vi "test bmp parse.vi"() -> ()   [LabVIEW 2018, in "Data Parser.lvclass"]
uses:
  Data Parser.lvclass
  Bmp data.ctl
panel:
  out "bmp data":T1
  in  "file string":string="<bmp\nname Rudolf\nhead sys/rudolf_f-r\nsmall sys/rudolf_s_x3\nfile(0-69) sys/rudolf-r_0 w 90 h 90 row 10 col 7\nfile(70-139) sys/rudolf-r_1 w 90 h 90 row 10 col 7\nfile(140-149) sys/rudolf-r_2 w 168 h 99 row 5 col 2\nfile(150-155) sys/rudolf-r_3 w 106 h 73 row 6 col 1\nwalking_frame_rate 3\nwalking_speed 6.000000\nwalking_speedz 2.500000\nrunning_frame_rate 3\nrunning_speed 13.000000\nrunning_speedz 1.600000\nheavy_walking_speed 4.200000\nheavy_walking_speedz 1.850000\nheavy_running_speed 7.000000\nheavy_running_speedz 1.000000\njump_height -16.299999\njump_distance 10.000000\njump_distancez 3.750000\ndash_height -10.000000\ndash_distance 18.000000\ndash_distancez 5.000000\nrowing_height -2.000000\nrowing_distance 5.000000\nlimb_head sys/limb_rudolf_head 1000 1000 5 5 0 25\nlimb_chest sys/limb_rudolf_chest 1000 1000 5 5 0 14\nlimb_hip sys/limb_rudolf_chest 1000 1000 5 5 20 17\nlimb_l_hand_a sys/limb_rudolf_hand 1000 1000 5 5 15 5\nlimb_r_hand_a sys/limb_rudolf_hand 1000 1000 5 5 25 4\nlimb_l_hand_b sys/limb_rudolf_hand 500 500 10 10 0 23\nlimb_r_hand_b sys/limb_rudolf_hand 500 500 10 10 30 23\nlimb_l_hand_w sys/limb_rudolf_weapon 1000 1000 5 5 0 5\nlimb_r_hand_w sys/limb_rudolf_weapon 1000 1000 5 5 0 5\nlimb_l_hand_c sys/limb_rudolf_hand_cover 500 500 10 10 0 23\nlimb_r_hand_c sys/limb_rudolf_hand_cover 500 500 10 10 30 23\nlimb_l_leg_a sys/limb_rudolf_leg 500 500 10 10 0 2\nlimb_l_leg_b sys/limb_rudolf_leg 500 500 10 10 10 6\nlimb_r_leg_a sys/limb_rudolf_leg 500 500 10 10 20 2\nlimb_r_leg_b sys/limb_rudolf_leg 500 500 10 10 30 6\nlimb_l_foot sys/limb_rudolf_leg 500 500 10 10 40 14\nlimb_r_foot sys/limb_rudolf_leg 500 500 10 10 60 14\nlimb_effect sys/limb_effect 1000 1000 5 5 0 25\nlimb_effect2 sys/limb_rudolf_effect 500 500 10 10 0 35\nlimb_head_blood 583 846 569 839 570 840 568 843 600 841 597 842 597 842 652 844 652 844 652 844 -1 -1 -1 -1 -1 -1 420 862 420 862 419 862 657 661 597 761 591 761 591 761 619 683 -1 -1 619 683 579 843 579 843 -1 -1 -1 -1 -1 -1 -1 -1 -1 -1\nlimb_hand_weapon 242 326 244 326 420 260 424 258 238 345 221 170 360 247 399 284 228 322 304 342 369 243 230 312 230 320 275 128 345 268 445 218 245 280 313 390 222 131 243 126 238 202 298 155 147 379 291 191 -1 -1 -1 -1 -1 -1 -1 -1 -1 -1 -1 -1 -1 -1 -1 -1 201 162 -1 -1 -1 -1 -1 -1 -1 -1 -1 -1 -1 -1 -1 -1 -1 -1 -1 -1 -1 -1 -1 -1 -1 -1 -1 -1 -1 -1 -1 -1 -1 -1 -1 -1 -1 -1 -1 -1 -1 -1 -1 -1 -1 -1 -1 -1 -1 -1 -1 -1 -1 -1 -1 -1\nresized 3\ndefault_centerx 44\ndefault_centery 84\nbmp>\n<f 0 standing\n   pic 0 wait 5 next 1 centerx 46 hit_Fa 285 hit_Fj 273 hit_Uj 250 hit_Dj 260 hit_ja 295\n   <bp x 48.464444444444446 y 38.35111111111111 bp>\n   <w kind 1 x 51 y 54 weaponact 30 cover 1 w>\n   <b kind 0 x 26 y 23 w 43 h 62 b>\nf>\n\n<f 1 -\n   pic 1 wait 4 next 2 dvz 123 centerx 47 hit_Fa 285 hit_Fj 273 hit_Uj 250 hit_Dj 260 hit_ja 295\n   <bp x 49.464444444444446 y 38.12888888888889 bp>\n   <w kind 1 x 52 y 54 weaponact 30 cover 1 w>\n   <b kind 0 x 26 y 23 w 43 h 62 b>\nf>\n\n<f 2 -\n   pic 2 wait 3 next 3 centerx 47 hit_Fa 285 hit_Fj 273 hit_Uj 250 hit_Dj 260 hit_ja 295\n   <bp x 49.464444444444446 y 37.906666666666666 bp>\n   <w kind 1 x 52 y 53 weaponact 30 cover 1 w>\n   <b kind 0 x 26 y 23 w 43 h 62 b>\nf>\n\n<f 3 -\n   pic 3 wait 8 next 4 hit_Fa 285 hit_Fj 273 hit_Uj 250 hit_Dj 260 hit_ja 295\n   <bp x 46.464444444444446 y 37.684444444444445 bp>\n   <w kind 1 x 49 y 52 weaponact 30 cover 1 w>\n   <b kind 0 x 26 y 23 w 43 h 62 b>\nf>\n\n<f 4 -\n   pic 2 wait 3 next 999 centerx 47 hit_Fa 285 hit_Fj 273 hit_Uj 250 hit_Dj 260 hit_ja 295\n   <bp x 49.464444444444446 y 37.906666666666666 bp>\n   <w kind 1 x 52 y 53 weaponact 30 cover 1 w>\n   <b kind 0 x 26 y 23 w 43 h 62 b>\nf>\n\n<f 5 walking\n   pic 4 state 1 wait 3 next 999 centerx 46 centery 83 hit_Fa 285 hit_Fj 273 hit_Uj 250 hit_Dj 260 hit_ja 295\n   <bp x 48.464444444444446 y 37.79555555555555 bp>\n   <w kind 1 x 49 y 51 weaponact 30 cover 1 w>\n   <i kind 1 x 45 y 21 w 25 h 65 catchingact 120 120 caughtact 130 130 i>\n   <b kind 0 x 27 y 18 w 34 h 64 b>\nf>\n\n<f 6 -\n   pic 5 state 1 wait 3 next 999 centerx 45 hit_Fa 285 hit_Fj 273 hit_Uj 250 hit_Dj 260 hit_ja 295\n   <bp x 47.464444444444446 y 38.79555555555555 bp>\n   <w kind 1 x 48 y 51 weaponact 30 cover 1 w>\n   <i kind 1 x 45 y 21 w 25 h 65 catchingact 120 120 caughtact 130 130 i>\n   <b kind 0 x 28 y 17 w 33 h 67 b>\nf>\n\n<f 7 -\n   pic 6 state 1 wait 3 next 999 centerx 47 hit_Fa 285 hit_Fj 273 hit_Uj 250 hit_Dj 260 hit_ja 295\n   <bp x 49.464444444444446 y 38.57333333333334 bp>\n   <w kind 1 x 50 y 51 weaponact 30 cover 1 w>\n   <i kind 1 x 45 y 21 w 25 h 65 catchingact 120 120 caughtact 130 130 i>\n   <b kind 0 x 29 y 16 w 34 h 67 b>\nf>\n\n<f 8 -\n   pic 7 state 1 wait 3 next 999 centerx 48 centery 83 hit_Fa 285 hit_Fj 273 hit_Uj 250 hit_Dj 260 hit_ja 295\n   <bp x 50.464444444444446 y 37.79555555555555 bp>\n   <w kind 1 x 52 y 51 weaponact 30 cover 1 w>\n   <i kind 1 x 45 y 21 w 25 h 65 catchingact 120 120 caughtact 130 130 i>\n   <b kind 0 x 31 y 17 w 34 h 65 b>\nf>\n\n<f 9 running\n   pic 20 state 2 wait 3 centerx 37\n   sound mp3/003\n   <bp x 65.5137545143159 y 55.18645971015323 bp>\n   <w kind 1 x 51 y 59 weaponact 32 cover 1 w>\n   <b kind 0 x 30 y 24 w 38 h 60 b>\nf>\n\n<f 10 -\n   pic 21 state 2 wait 3 centerx 37\n   <bp x 65.5137545143159 y 56.29757082126433 bp>\n   <w kind 1 x 51 y 60 weaponact 32 cover 1 w>\n   <b kind 0 x 30 y 24 w 38 h 60 b>\nf>\n\n<f 11 -\n   pic 22 state 2 wait 3 centerx 37\n   sound mp3/004\n   <bp x 65.5137545143159 y 55.18645971015323 bp>\n   <w kind 1 x 51 y 61 weaponact 32 cover 1 w>\n   <b kind 0 x 30 y 24 w 38 h 60 b>\nf>\n\n<f 12 heavy_obj_walk\n   pic 23 state 1 wait 3 centerx 45\n   <bp x 46.79777777777778 y 39.24 bp>\n   <w kind 1 x 42.22222222222222 y 24.875555555555557 weaponact 10 w>\n   <b kind 0 x 26 y 17 w 38 h 71 b>\nf>\n\n<f 13 -\n   pic 24 state 1 wait 3\n   <bp x 45.79777777777778 y 39.01777777777778 bp>\n   <w kind 1 x 41.22222222222222 y 24.653333333333336 weaponact 10 w>\n   <b kind 0 x 27 y 18 w 36 h 69 b>\nf>\n\n<f 14 -\n   pic 25 state 1 wait 3 centerx 46\n   <bp x 47.79777777777778 y 39.01777777777778 bp>\n   <w kind 1 x 43.22222222222222 y 24.653333333333336 weaponact 10 w>\n   <b kind 0 x 27 y 16 w 38 h 70 b>\nf>\n\n<f 15 -\n   pic 26 state 1 wait 3 centerx 48\n   <bp x 49.79777777777778 y 38.79555555555555 bp>\n   <w kind 1 x 45.22222222222222 y 24.431111111111115 weaponact 10 w>\n   <b kind 0 x 29 y 16 w 38 h 72 b>\nf>\n\n<f 16 heavy_obj_run\n   pic 125 state 2 wait 3 centerx 40\n   sound mp3/003\n   <bp x 41.79777777777778 y 38.79555555555555 bp>\n   <w kind 1 x 37.22222222222222 y 24.431111111111115 weaponact 10 w>\n   <b kind 0 x 27 y 15 w 30 h 68 b>\nf>\n\n<f 17 -\n   pic 126 state 2 wait 3\n   <bp x 45.79777777777778 y 38.35111111111111 bp>\n   <w kind 1 x 41.22222222222222 y 23.986666666666665 weaponact 10 w>\n   <b kind 0 x 33 y 15 w 31 h 68 b>\nf>\n\n<f 18 -\n   pic 127 state 2 wait 3 centerx 46\n   sound mp3/004\n   <bp x 47.79777777777778 y 38.79555555555555 bp>\n   <w kind 1 x 43.22222222222222 y 24.653333333333336 weaponact 10 w>\n   <b kind 0 x 29 y 20 w 37 h 63 b>\nf>\n\n<f 19 heavy_stop_run\n   pic 128 state 15 wait 7 next 999 dvx 2 centerx 38\n   sound mp3/009\n   <bp x 41.32306886667164 y 39.190553757669235 bp>\n   <w kind 1 x 38.8899896983711 y 24.335554073121564 weaponact 10 w>\n   <b kind 0 x 23 y 21 w 38 h 63 b>\nf>\n\n<f 20 normal_weapon_atck\n   pic 70 state 3 wait 1 next 21 centerx 38\n   <bp x 39.8 y 37.82222222222222 bp>\n   <w kind 1 x 26.592545073322224 y 22.254645252289063 weaponact 31 w>\n   <b kind 0 x 26 y 19 w 34 h 65 b>\nf>\n\n<f 21 -\n   pic 71 state 3 wait 1 next 22 centerx 38\n   sound mp3/008\n   <bp x 43.62444444444444 y 37.92444444444445 bp>\n   <w kind 1 x 41.63440528554246 y 21.504109467745614 weaponact 32 w>\n   <b kind 0 x 29 y 17 w 28 h 67 b>\nf>\n\n<f 22 -\n   pic 72 state 3 wait 1 next 23 centerx 33\n   <bp x 44.08982646609609 y 39.58924737843303 bp>\n   <w kind 1 x 49.32160589714093 y 59.440946875407946 weaponact 24 attacking 1 w>\n   <b kind 0 x 12 y 17 w 40 h 68 b>\nf>\n\n<f 23 -\n   pic 73 state 3 wait 1 next 999 centerx 33 centery 85\n   <bp x 46.58183747280419 y 41.68501265613956 bp>\n   <w kind 1 x 41.82331609590126 y 64.18428829073993 weaponact 25 w>\n   <b kind 0 x 14 y 17 w 34 h 69 b>\n   <b kind 0 x 30 y 66 w 17 h 18 b>\nf>\n\n<f 25 normal_weapon_atck\n   pic 74 state 3 wait 1 next 26 centerx 41\n   <bp x 50.17696571753358 y 39.06775950420733 bp>\n   <w kind 1 x 52 y 51 weaponact 33 cover 1 w>\n   <b kind 0 x 24 y 13 w 33 h 72 b>\nf>\n\n<f 26 -\n   pic 75 state 3 wait 1 next 27 centerx 41\n   sound mp3/008\n   <bp x 49.07477201946767 y 38.68260033531007 bp>\n   <w kind 1 x 58 y 47 weaponact 32 cover 1 w>\n   <b kind 0 x 29 y 17 w 27 h 67 b>\nf>\n\n<f 27 -\n   pic 76 state 3 wait 1 next 28 centerx 33\n   <bp x 39.39302438590751 y 39.56103447170426 bp>\n   <w kind 1 x 50.64327642640106 y 56.22124561746575 weaponact 24 attacking 1 w>\n   <b kind 0 x 14 y 20 w 32 h 64 b>\nf>\n\n<f 28 -\n   pic 77 state 3 wait 1 next 999\n   <bp x 56.25248349990373 y 42.434129183191274 bp>\n   <w kind 1 x 26.13347160923185 y 54.783390010013164 weaponact 25 w>\n   <b kind 0 x 29 y 23 w 32 h 60 b>\nf>\n\n<f 30 jump_weapon_atck\n   pic 80 state 3 wait 1 next 31 centerx 29 centery 89\n   <bp x 41.46019077473909 y 38.358365142781864 bp>\n   <w kind 1 x 29.95234256553649 y 21.49551402119002 weaponact 32 w>\n   <b kind 0 x 21 y 18 w 28 h 58 b>\nf>\n\n<f 31 -\n   pic 81 state 3 wait 1 next 32 centerx 27 centery 90\n   sound mp3/008\n   <bp x 42.49276045988708 y 39.645255650438315 bp>\n   <w kind 1 x 42.23001532517321 y 23.106857251707368 weaponact 33 attacking 2 w>\n   <b kind 0 x 28 y 15 w 23 h 45 b>\n   <b kind 0 x 18 y 43 w 24 h 33 b>\nf>\n\n<f 32 -\n   pic 82 state 3 wait 1 next 33 centerx 25 centery 91\n   <bp x 44.97871535498498 y 41.478136267321915 bp>\n   <w kind 1 x 50.97547888680435 y 60.889746033215864 weaponact 24 attacking 2 w>\n   <b kind 0 x 16 y 37 w 33 h 43 b>\n   <b kind 0 x 34 y 17 w 26 h 38 b>\nf>\n\n<f 33 -\n   pic 83 state 3 wait 4 next 999 centerx 27 centery 92\n   <bp x 47.24850413947085 y 43.129457100584006 bp>\n   <w kind 1 x 42.489982762567934 y 65.62873273518439 weaponact 25 attacking 2 w>\n   <b kind 0 x 16 y 37 w 33 h 43 b>\n   <b kind 0 x 31 y 14 w 26 h 37 b>\nf>\n\n<f 35 run_weapon_atck\n   pic 71 state 3 wait 1 next 36 dvx 6 centerx 45\n   <bp x 43.62444444444444 y 37.92444444444445 bp>\n   <w kind 1 x 41.63440528554246 y 21.504109467745614 weaponact 32 w>\n   <b kind 0 x 26 y 20 w 31 h 65 b>\nf>\n\n<f 36 -\n   pic 72 state 3 wait 1 next 37 dvx 4 centerx 31\n   sound mp3/008\n   <bp x 44.08982646609609 y 39.58924737843303 bp>\n   <w kind 1 x 49.32160589714093 y 58.440946875407946 weaponact 23 attacking 3 w>\n   <b kind 0 x 20 y 20 w 29 h 63 b>\nf>\n\n<f 37 -\n   pic 73 wait 6 next 999 centerx 29\n   <bp x 46.58183747280419 y 41.68501265613956 bp>\n   <w kind 1 x 42.82331609590126 y 64.18428829073993 weaponact 24 attacking 3 w>\n   <b kind 0 x 22 y 22 w 26 h 61 b>\nf>\n\n<f 40 dash_weapon_atck\n   pic 80 state 3 wait 1 next 41 centerx 26 centery 82\n   <bp x 41.46019077473909 y 38.358365142781864 bp>\n   <w kind 1 x 29.95234256553649 y 21.49551402119002 weaponact 31 w>\n   <b kind 0 x 20 y 20 w 27 h 56 b>\nf>\n\n<f 41 -\n   pic 81 state 3 wait 1 next 42 centerx 25 centery 83\n   sound mp3/008\n   <bp x 42.49276045988708 y 39.645255650438315 bp>\n   <w kind 1 x 42.23001532517321 y 23.106857251707368 weaponact 33 attacking 4 w>\n   <b kind 0 x 13 y 37 w 33 h 45 b>\n   <b kind 0 x 28 y 13 w 34 h 33 b>\nf>\n\n<f 42 -\n   pic 82 state 3 wait 1 next 43 centerx 23 centery 83\n   <bp x 44.97871535498498 y 41.478136267321915 bp>\n   <w kind 1 x 51.97547888680435 y 60.889746033215864 weaponact 24 attacking 4 w>\n   <b kind 0 x 13 y 37 w 33 h 45 b>\n   <b kind 0 x 32 y 18 w 30 h 33 b>\nf>\n\n<f 43 -\n   pic 83 state 3 wait 8 next 999 centerx 25\n   <bp x 47.24850413947085 y 43.129457100584006 bp>\n   <w kind 1 x 42.489982762567934 y 64.62873273518439 weaponact 25 attacking 4 w>\n   <b kind 0 x 13 y 37 w 33 h 45 b>\n   <b kind 0 x 28 y 18 w 31 h 37 b>\nf>\n\n<f 45 light_weapon_thw\n   pic 94 state 15 wait 3 next 46\n   <bp x 44.846666666666664 y 38.59111111111111 bp>\n   <w kind 1 x 42.85662750776468 y 22.17077613441228 weaponact 32 w>\n   <b kind 0 x 24 y 20 w 34 h 65 b>\nf>\n\n<f 46 -\n   pic 95 state 15 wait 1 next 47 centerx 42\n   sound mp3/008\n   <bp x 49.31204868831831 y 40.478136267321915 bp>\n   <w kind 1 x 58.535850652335206 y 58.54142301823171 weaponact 22 w>\n   <b kind 0 x 29 y 27 w 32 h 57 b>\nf>\n\n<f 47 -\n   pic 96 state 15 wait 9 next 999 centerx 35\n   <w kind 1 x 107 y 65 weaponact 35 dvx 19 dvy -4 dvz 3 w>\n   <b kind 0 x 15 y 43 w 54 h 21 b>\n   <b kind 0 x 31 y 60 w 32 h 26 b>\nf>\n\n<f 50 heavy_weapon_thw\n   pic 27 state 15 wait 4 next 51\n   <bp x 44.53670834964537 y 38.96496959566491 bp>\n   <w kind 1 x 39.986319716818436 y 25.419297977363684 weaponact 10 w>\n   <b kind 0 x 23 y 19 w 37 h 66 b>\nf>\n\n<f 51 -\n   pic 28 state 15 wait 7 next 999 centerx 39\n   sound mp3/007\n   <w kind 1 x 104 y 47 weaponact 10 dvx 9 dvy -4 dvz 2 w>\n   <b kind 0 x 13 y 44 w 61 h 23 b>\n   <b kind 0 x 26 y 27 w 39 h 57 b>\nf>\n\n<f 52 sky_lgt_wp_thw\n   pic 97 state 15 wait 3 next 53 centerx 29 centery 76\n   <bp x 44.46019077473909 y 32.35836514278185 bp>\n   <w kind 1 x 32.9523425655365 y 14.49551402119002 weaponact 31 w>\n   <b kind 0 x 26 y 17 w 34 h 52 b>\nf>\n\n<f 53 -\n   pic 98 state 15 wait 1 next 54 dvy -2 centerx 30 centery 77\n   sound mp3/008\n   <bp x 47.49276045988708 y 33.64525565043831 bp>\n   <w kind 1 x 47.23001532517321 y 17.106857251707368 weaponact 34 w>\n   <b kind 0 x 25 y 12 w 31 h 66 b>\nf>\n\n<f 54 -\n   pic 99 state 15 wait 9 next 999 centerx 33 centery 76\n   <w kind 1 x 80 y 70 weaponact 23 dvx 16 dvy 8 dvz 3 w>\n   <b kind 0 x 32 y 27 w 36 h 34 b>\n   <b kind 0 x 8 y 42 w 34 h 26 b>\nf>\n\n<f 55 weapon_drink\n   pic 105 state 17 wait 3 next 56 centerx 45 hit_d 999\n   sound mp3/042\n   <w kind 1 x 62.950240476147165 y 27.81086947083836 weaponact 31 w>\n   <b kind 0 x 20 y 17 w 37 h 67 b>\nf>\n\n<f 56 -\n   pic 106 state 17 wait 3 next 57 centerx 45 hit_d 999\n   <w kind 1 x 62.80507006707795 y 26.583434474775675 weaponact 31 w>\n   <b kind 0 x 21 y 25 w 36 h 59 b>\nf>\n\n<f 57 -\n   pic 107 state 17 wait 3 next 58 centerx 45 hit_d 999\n   <w kind 1 x 62.80507006707795 y 25.91676780810901 weaponact 31 w>\n   <b kind 0 x 22 y 22 w 32 h 63 b>\nf>\n\n<f 58 -\n   pic 106 state 17 wait 3 next 55 centerx 45 hit_d 999\n   <w kind 1 x 62.80507006707795 y 26.583434474775675 weaponact 31 w>\n   <b kind 0 x 21 y 18 w 36 h 65 b>\nf>\n\n<f 59 punch\n   pic 13 state 3 wait 4 next 999 centerx 46\n   <bp x 51.45702584630638 y 39.20820242827308 bp>\n   <b kind 0 x 29 y 18 w 33 h 66 b>\nf>\n\n<f 60 -\n   pic 10 state 3 wait 3 next 61 centerx 45 mp 15\n   <bp x 48.75061461791846 y 38.42940829813039 bp>\n   <i kind 2 x 26 y 62 w 37 h 24 vrest 1 i>\n   <b kind 0 x 28 y 20 w 31 h 63 b>\nf>\n\n<f 61 -\n   pic 11 state 3 wait 2 next 62 centerx 47\n   sound mp3/007\n   <bp x 51.18 y 38.59111111111111 bp>\n   <b kind 0 x 33 y 19 w 29 h 63 b>\nf>\n\n<f 62 -\n   pic 12 state 3 wait 1 next 63 centerx 45\n   <o kind 1 x 80 y 62 action 40 dvx 19 dvy -3 oid 202 o>\n   <bp x 49.825838059315736 y 38.98216753134385 bp>\n   <b kind 0 x 31 y 21 w 30 h 64 b>\nf>\n\n<f 63 -\n   pic 13 state 3 wait 4 next 999 centerx 46 hit_a 64\n   <bp x 51.45702584630638 y 39.20820242827308 bp>\n   <b kind 0 x 28 y 17 w 32 h 69 b>\nf>\n\n<f 64 -\n   pic 14 state 3 wait 2 next 66 centerx 47 mp 15\n   <bp x 51.18 y 38.59111111111111 bp>\n   <b kind 0 x 29 y 17 w 30 h 66 b>\nf>\n\n<f 65 -\n   pic 10 state 3 wait 3 next 61 centerx 45 mp 15\n   <bp x 48.75061461791846 y 38.42940829813039 bp>\n   <i kind 2 x 26 y 62 w 37 h 24 vrest 1 i>\n   <b kind 0 x 27 y 23 w 32 h 60 b>\nf>\n\n<f 66 -\n   pic 15 state 3 wait 3 next 67 centerx 45\n   <o kind 1 x 80 y 62 action 40 dvx 18 dvy -2 oid 202 o>\n   <bp x 50.45702584630638 y 39.20820242827308 bp>\n   <b kind 0 x 29 y 20 w 30 h 65 b>\nf>\n\n<f 67 -\n   pic 13 state 3 wait 1 next 999 centerx 46 hit_a 68\n   <bp x 51.45702584630638 y 39.20820242827308 bp>\n   <b kind 0 x 33 y 20 w 27 h 64 b>\nf>\n\n<f 68 -\n   pic 14 state 3 wait 2 next 69 centerx 47 mp 15\n   <bp x 51.18 y 38.59111111111111 bp>\n   <b kind 0 x 32 y 20 w 32 h 62 b>\nf>\n\n<f 69 -\n   pic 12 state 3 wait 2 next 59 centerx 45\n   <o kind 1 x 80 y 62 action 40 dvx 17 dvy -1 oid 202 o>\n   <bp x 49.825838059315736 y 38.98216753134385 bp>\n   <b kind 0 x 30 y 18 w 32 h 66 b>\nf>\n\n<f 70 super_punch\n   pic 132 state 3 wait 1 next 71 centerx 35\n   <bp x 39.18 y 39.257777777777775 bp>\n   <b kind 0 x 19 y 19 w 30 h 66 b>\nf>\n\n<f 71 -\n   pic 133 state 3 wait 2 next 72 dvx 4 centerx 32\n   sound mp3/028\n   <bp x 37.78915887559496 y 40.08682004994553 bp>\n   <i kind 0 x 50 y 14 w 36 h 51 dvx -3 dvy -4 fall 1 injury 10 effect 1 i>\n   <b kind 0 x 9 y 21 w 39 h 61 b>\nf>\n\n<f 72 -\n   pic 134 state 3 wait 1 next 73\n   <i kind 0 x 4 y 11 w 76 h 36 dvx -3 dvy -4 fall 1 injury 10 effect 1 i>\n   <b kind 0 x 27 y 22 w 28 h 62 b>\nf>\n\n<f 73 -\n   pic 135 state 3 wait 1 next 74 centerx 50\n   <b kind 0 x 31 y 19 w 31 h 64 b>\nf>\n\n<f 74 -\n   pic 136 state 3 wait 2 next 75 centerx 37\n   sound mp3/029\n   <bp x 40.933663000829135 y 40.21290188827957 bp>\n   <i kind 0 x 51 y 18 w 32 h 64 dvx 7 dvy -4 fall 70 bdefend 60 injury 65 effect 1 i>\n   <b kind 0 x 18 y 19 w 29 h 64 b>\nf>\n\n<f 75 -\n   pic 137 state 3 wait 1 next 76 centerx 43 centery 82\n   <bp x 45.328713933213194 y 38.15890324252262 bp>\n   <i kind 0 x 5 y 52 w 62 h 31 dvx 7 dvy -4 fall 70 bdefend 60 injury 65 effect 1 i>\n   <b kind 0 x 19 y 14 w 39 h 70 b>\nf>\n\n<f 76 -\n   pic 138 state 3 wait 1 next 77 centerx 49 centery 81\n   <bp x 51.10649171099097 y 37.15890324252262 bp>\n   <b kind 0 x 27 y 16 w 39 h 67 b>\nf>\n\n<f 77 -\n   pic 139 state 3 wait 2 next 78 centerx 55 centery 83\n   <bp x 56.88426948876875 y 39.15890324252262 bp>\n   <b kind 0 x 32 y 18 w 39 h 66 b>\nf>\n\n<f 78 -\n   pic 129 state 3 wait 2 next 79 centerx 48 centery 83\n   <b kind 0 x 27 y 22 w 46 h 63 b>\nf>\n\n<f 79 -\n   pic 119 state 3 wait 3 next 999 centerx 47 centery 83\n   sound mp3/027\n   <bp x 54.268509856829496 y 38.507330714964766 bp>\n   <b kind 0 x 26 y 20 w 42 h 64 b>\nf>\n\n<f 80 jump_attack\n   pic 67 state 3 wait 1 next 81 centerx 38 centery 83\n   <bp x 42.18 y 38.257777777777775 bp>\n   <b kind 0 x 32 y 17 w 30 h 63 b>\nf>\n\n<f 81 -\n   pic 68 state 3 wait 1 next 82 centerx 34 centery 83\n   sound mp3/028\n   <bp x 39.78915887559496 y 39.08682004994553 bp>\n   <i kind 0 x 43 y 13 w 53 h 40 dvx -2 dvy -2 fall 20 arest 15 bdefend 60 injury 35 effect 1 i>\n   <b kind 0 x 24 y 20 w 34 h 60 b>\nf>\n\n<f 82 -\n   pic 69 state 3 wait 1 next 83 centerx 43 centery 82\n   <i kind 0 x 11 y 7 w 75 h 22 dvx -2 dvy -2 fall 20 arest 15 bdefend 60 injury 35 effect 1 i>\n   <b kind 0 x 31 y 18 w 32 h 64 b>\nf>\n\n<f 83 -\n   pic 29 state 3 wait 1 next 84 centerx 51 centery 82\n   <b kind 0 x 38 y 11 w 35 h 70 b>\nf>\n\n<f 84 -\n   pic 39 state 3 wait 1 next 118 centerx 41\n   sound mp3/029\n   <bp x 44.933663000829135 y 40.21290188827957 bp>\n   <i kind 0 x 58 y 11 w 37 h 62 dvx 1 fall 60 arest 15 bdefend 60 injury 35 effect 1 i>\n   <b kind 0 x 26 y 13 w 34 h 67 b>\nf>\n\n<f 85 run_attack\n   pic 140 state 3 wait 1 next 86 dvx 12 centerx 45 centery 90\n   <bp x 73.51375451431592 y 61.18645971015323 bp>\n   <b kind 0 x 30 y 39 w 50 h 52 b>\nf>\n\n<f 86 -\n   pic 141 state 3 wait 1 next 87 dvx 12 centerx 37 centery 90\n   sound mp3/029\n   <i kind 0 x 65 y 36 w 66 h 48 dvx -4 dvy -4 injury 45 effect 1 i>\n   <b kind 0 x 23 y 38 w 49 h 51 b>\nf>\n\n<f 87 -\n   pic 142 state 3 wait 1 next 88 centerx 48 centery 90\n   sound mp3/028\n   <bp x 75.91504918785502 y 61.27127540437745 bp>\n   <i kind 0 x 65 y 36 w 66 h 48 dvx -4 dvy -4 injury 45 effect 1 i>\n   <b kind 0 x 30 y 39 w 51 h 48 b>\nf>\n\n<f 88 -\n   pic 143 state 3 wait 1 next 89 centerx 53 centery 90\n   <bp x 80.47060474341058 y 60.82683095993299 bp>\n   <i kind 0 x 22 y 35 w 81 h 53 dvx 10 dvy -7 fall 70 vrest 15 bdefend 60 injury 35 effect 1 i>\n   <b kind 0 x 36 y 39 w 49 h 52 b>\nf>\n\n<f 89 -\n   pic 144 state 3 wait 6 next 78 centerx 57 centery 90\n   <bp x 84.24838252118836 y 60.82683095993299 bp>\n   <b kind 0 x 41 y 41 w 45 h 49 b>\nf>\n\n<f 90 dash_attack\n   pic 145 state 3 wait 1 next 91 centerx 45 centery 90\n   <bp x 73.51375451431592 y 61.18645971015323 bp>\n   <b kind 0 x 30 y 39 w 50 h 52 b>\nf>\n\n<f 91 -\n   pic 146 state 3 wait 1 next 92 centerx 50 centery 90\n   sound mp3/029\n   <b kind 0 x 38 y 33 w 53 h 52 b>\nf>\n\n<f 92 -\n   pic 147 state 3 wait 1 next 93 centerx 49 centery 90\n   sound mp3/028\n   <bp x 76.91504918785502 y 61.27127540437745 bp>\n   <i kind 0 x 62 y 29 w 54 h 55 dvx 10 dvy -7 fall 70 vrest 15 bdefend 60 injury 75 effect 1 i>\n   <b kind 0 x 30 y 39 w 51 h 48 b>\nf>\n\n<f 93 -\n   pic 148 state 3 wait 1 next 94 centerx 53 centery 90\n   <bp x 80.47060474341058 y 60.82683095993299 bp>\n   <i kind 0 x 62 y 29 w 54 h 55 dvx 10 dvy -7 fall 70 vrest 15 bdefend 60 injury 75 effect 1 i>\n   <b kind 0 x 36 y 39 w 49 h 52 b>\nf>\n\n<f 94 -\n   pic 149 state 3 wait 6 centerx 48 centery 90\n   <bp x 75.24838252118836 y 60.82683095993299 bp>\n   <b kind 0 x 41 y 41 w 45 h 49 b>\nf>\n\n<f 95 dash_defend\n   pic 0 state 7 wait 2\n   <w kind 1 x 26 y 32 weaponact 30 w>\n   <b kind 0 x 19 y 24 w 28 h 36 b>\n   <b kind 0 x 33 y 42 w 24 h 34 b>\nf>\n\n<f 100 rowing\n   pic 66 state 6 wait 2 next 101\n   sound mp3/017\n   <w kind 1 x 41 y 47 weaponact 32 cover 1 w>\nf>\n\n<f 101 -\n   pic 65 state 6 wait 6\n   <w kind 1 x 43.95170419050154 y 78.63834992199499 weaponact 24 w>\nf>\n\n<f 102 -\n   pic 16 state 6 wait 1 next 103 dvx 12 hit_Fj 274\n   sound mp3/030\n   <w kind 1 x 49 y 62 weaponact 32 cover 1 w>\nf>\n\n<f 103 -\n   pic 17 state 6 wait 1 next 104 dvx 12 centery 85 hit_Fj 274\n   <w kind 1 x 50 y 62 weaponact 32 cover 1 w>\nf>\n\n<f 104 -\n   pic 37 state 6 wait 4 next 105 dvx 15 hit_Fj 274\n   <w kind 1 x 54 y 62 weaponact 32 cover 1 w>\nf>\n\n<f 105 -\n   pic 37 state 6 wait 1 next 106 dvx 15 hit_Fj 274\n   <w kind 1 x 54 y 61 weaponact 32 cover 1 w>\nf>\n\n<f 106 -\n   pic 18 state 6 wait 1 next 219 hit_Fj 274\n   <w kind 1 x 55 y 62 weaponact 32 cover 1 w>\nf>\n\n<f 107 -\n   pic 19 state 6 wait 1 next 219 hit_Fj 274\n   <w kind 1 x 52 y 62 weaponact 32 cover 1 w>\nf>\n\n<f 108 -\n   pic 117 state 6 wait 3 next 109 centerx 50 centery 67 hit_Fj 274\n   sound mp3/017\n   <w kind 1 x 34.04076445853931 y 54.321495573617526 weaponact 34 w>\nf>\n\n<f 109 -\n   pic 118 state 6 wait 6 hit_Fj 274\n   <bp x 49.25902051805167 y 33.144509517513825 bp>\n   <w kind 1 x 25.2908229291307 y 49.8899842303862 weaponact 25 w>\nf>\n\n<f 110 defend\n   pic 56 state 7 wait 12 next 999 centerx 33 hit_Fa 285 hit_Fj 273 hit_Uj 250 hit_Dj 260 hit_ja 295\n   <bp x 39.94688433155981 y 39.83457848056723 bp>\n   <w kind 1 x 44 y 56 weaponact 31 cover 1 w>\n   <b kind 0 x 25 y 24 w 38 h 60 b>\nf>\n\n<f 111 -\n   pic 57 state 7 next 110 centerx 40\n   <bp x 48.80024533612795 y 40.97072258580963 bp>\n   <w kind 1 x 50 y 56 weaponact 31 cover 1 w>\n   <b kind 0 x 21 y 24 w 42 h 60 b>\nf>\n\n<f 112 broken_defend\n   pic 46 state 8 wait 2 next 113 dvx -2\n   <bp x 33.61747589432981 y 43.877840195795926 bp>\n   <w kind 1 x 44 y 56 weaponact 31 cover 1 w>\n   <i kind 6 x -4 y 21 w 85 h 65 vrest 1 i>\n   <b kind 0 x 10 y 22 w 64 h 65 b>\nf>\n\n<f 113 -\n   pic 47 state 8 wait 2 next 114 dvx -2\n   <bp x 32.834483274563965 y 45.21877792596001 bp>\n   <w kind 1 x 45 y 55 weaponact 31 cover 1 w>\n   <i kind 6 x -4 y 21 w 85 h 65 vrest 1 i>\n   <b kind 0 x 10 y 22 w 64 h 65 b>\nf>\n\n<f 114 -\n   pic 48 state 8 wait 2 next 999 dvx -2\n   <bp x 31.699668361400455 y 41.62497029228115 bp>\n   <w kind 1 x 43 y 56 weaponact 31 cover 1 w>\n   <i kind 6 x -4 y 21 w 85 h 65 vrest 1 i>\n   <b kind 0 x 10 y 22 w 64 h 65 b>\nf>\n\n<f 115 picking_light\n   pic 36 state 15 wait 4 next 999\n   sound mp3/009\n   <bp x 46.1008823727453 y 52.92179047137672 bp>\n   <w kind 1 x 31 y 80 weaponact 24 w>\n   <b kind 0 x 27 y 35 w 33 h 49 b>\nf>\n\n<f 116 picking_heavy\n   pic 36 state 15 wait 2 next 117\n   sound mp3/009\n   <w kind 1 x 46 y 84 weaponact 10 w>\n   <b kind 0 x 30 y 32 w 31 h 52 b>\nf>\n\n<f 117 -\n   pic 36 state 15 wait 2 next 999\n   <w kind 1 x 46 y 80 weaponact 10 w>\n   <b kind 0 x 30 y 35 w 33 h 48 b>\nf>\n\n<f 118 jump_attack\n   pic 49 state 3 wait 1 next 119 centerx 45 centery 83\n   <bp x 47.328713933213194 y 39.15890324252262 bp>\n   <i kind 0 x 13 y 44 w 67 h 38 dvx 1 fall 60 arest 15 bdefend 60 injury 35 effect 1 i>\n   <b kind 0 x 26 y 13 w 37 h 68 b>\nf>\n\n<f 119 -\n   pic 59 state 3 wait 12 next 999 centerx 51 centery 83\n   <bp x 53.10649171099097 y 39.15890324252262 bp>\n   <b kind 0 x 32 y 13 w 39 h 71 b>\nf>\n\n<f 120 catching\n   pic 51 state 9 wait 2 next 121 centerx 43\n   sound mp3/015\n   <bp x 50.36526968138738 y 40.172935507380345 bp>\n   <c kind 1 x 72 y 44 vaction 131 hurtable 1 decrease 7 c>\n   <w kind 1 x 45 y 54 weaponact 31 cover 1 w>\n   <b kind 0 x 24 y 20 w 28 h 65 b>\nf>\n\n<f 121 -\n   pic 50 state 9 hit_ja 235\n   <bp x 53.5874919036096 y 40.172935507380345 bp>\n   <c kind 1 x 66 y 44 vaction 130 aaction 122 taction -232 hurtable 1 decrease -7 c>\n   <w kind 1 x 50 y 54 weaponact 31 cover 1 w>\n   <b kind 0 x 24 y 20 w 28 h 65 b>\nf>\n\n<f 122 -\n   pic 51 state 9 wait 5 next 123 centerx 43\n   <bp x 50.36526968138738 y 40.172935507380345 bp>\n   <c kind 1 x 66 y 44 vaction 130 hurtable 1 decrease 7 c>\n   <w kind 1 x 46 y 54 weaponact 31 cover 1 w>\n   <b kind 0 x 24 y 20 w 28 h 65 b>\nf>\n\n<f 123 -\n   pic 52 state 9 wait 3 next 121\n   sound mp3/014\n   <bp x 54.39766238486479 y 40.49462534986445 bp>\n   <c kind 1 x 63 y 43 injury 15 vaction 132 hurtable 1 decrease 3 c>\n   <w kind 1 x 48 y 53 weaponact 31 cover 1 w>\n   <b kind 0 x 24 y 20 w 28 h 65 b>\nf>\n\n<f 130 picked_caught\n   pic 53 state 10 wait 3\n   <bp x 40.622517564109046 y 34.00226443970676 bp>\n   <c kind 2 x 47 y 44 fronthurtact 132 backhurtact 131 c>\n   <w kind 1 x 36.9997312660619 y 57.89388139500498 weaponact 25 w>\n   <b kind 0 x 31 y 19 w 28 h 66 b>\nf>\n\n<f 131 -\n   pic 54 state 10 wait 3\n   <bp x 41.77333743822034 y 33.66075076504629 bp>\n   <c kind 2 x 48 y 44 fronthurtact 132 backhurtact 132 c>\n   <w kind 1 x 41.1675015423386 y 57.803519072722274 weaponact 26 w>\n   <b kind 0 x 31 y 19 w 28 h 66 b>\nf>\n\n<f 132 -\n   pic 55 state 10 wait 3\n   <bp x 54.11630841755195 y 42.5521665331587 bp>\n   <c kind 2 x 46 y 44 fronthurtact 131 backhurtact 131 c>\n   <w kind 1 x 41.51353026324553 y 57.455376480517536 weaponact 26 w>\n   <b kind 0 x 31 y 19 w 28 h 66 b>\nf>\n\n<f 133 -\n   pic 30 state 10 wait 3\n   <bp x 42.499641877617954 y 42.65335136303321 bp>\n   <c kind 2 x 38 y 41 c>\n   <w kind 1 x 36.381704779300506 y 54.713175825347946 weaponact 22 w>\nf>\n\n<f 134 -\n   pic 31 state 10 wait 3 centerx 45\n   <bp x 29.30119872526209 y 28.79651920190857 bp>\n   <c kind 2 x 37 y 40 c>\n   <w kind 1 x 43.77779948258218 y 39.055331510048525 weaponact 21 w>\nf>\n\n<f 135 -\n   pic 32 state 10 wait 3\n   <bp x 29.625771905318558 y 31.904352557110816 bp>\n   <c kind 2 x 43 y 38 c>\n   <w kind 1 x 51.19999790204919 y 41.1208037036435 weaponact 21 w>\nf>\n\n<f 136 -\n   pic 33 state 10 wait 3\n   <c kind 2 x 39 y 49 c>\n   <w kind 1 x 41 y 43 weaponact 33 cover 1 w>\nf>\n\n<f 137 -\n   pic 34 state 10 wait 3 centery 76\n   <bp x 29.353407673173237 y 64.34448184526693 bp>\n   <c kind 2 x 41 y 73 c>\n   <w kind 1 x 51.71790734309482 y 78.66647331391574 weaponact 32 w>\nf>\n\n<f 138 -\n   pic 35 state 10 wait 3\n   <bp x 30.190230589916823 y 50.830624988374424 bp>\n   <c kind 2 x 39 y 59 c>\n   <w kind 1 x 42.150696657273585 y 74.69644233620875 weaponact 31 w>\nf>\n\n<f 139 -\n   pic 40 state 10 wait 3\n   <bp x 44.3164372178733 y 27.33384943352798 bp>\n   <c kind 2 x 45 y 41 c>\n   <w kind 1 x 38.345639099432866 y 53.21421790570382 weaponact 35 w>\nf>\n\n<f 140 -\n   pic 41 state 10 wait 3\n   <bp x 51.38853076650684 y 42.65335136303321 bp>\n   <c kind 2 x 41 y 43 c>\n   <w kind 1 x 32.76090299281674 y 51.4072386275756 weaponact 20 w>\nf>\n\n<f 141 -\n   pic 42 state 10 wait 3\n   <bp x 56.74213190441054 y 51.00492542155155 bp>\n   <c kind 2 x 49 y 45 c>\n   <w kind 1 x 50.35173633117958 y 62.1625229218968 weaponact 23 w>\nf>\n\n<f 142 -\n   pic 43 state 10 wait 3\n   <bp x 56.2976874599661 y 66.5604809771071 bp>\n   <c kind 2 x 51 y 56 c>\n   <w kind 1 x 50.35173633117958 y 73.27363403300791 weaponact 25 w>\nf>\n\n<f 143 -\n   pic 44 state 10 wait 3 centery 79\n   <bp x 57.4138808745262 y 81.81636069893024 bp>\n   <c kind 2 x 50 y 71 c>\n   <w kind 1 x 48.43042360707956 y 82.3016868465666 weaponact 24 w>\nf>\n\n<f 144 -\n   pic 45 state 10 wait 3\n   <bp x 56.74213190441054 y 57.67159208821822 bp>\n   <c kind 2 x 47 y 60 c>\n   <w kind 1 x 50.35173633117958 y 68.82918958856347 weaponact 25 w>\nf>\n\n<f 180 falling\n   pic 30 state 12 wait 3\n   <bp x 42.499641877617954 y 42.65335136303321 bp>\n   <w kind 1 x 36.381704779300506 y 54.713175825347946 weaponact 21 w>\n   <i kind 4 x 26 y 19 w 29 h 44 dvx 2 fall 70 vrest 20 bdefend 10 injury 30 i>\n   <b kind 0 x 30 y 30 w 21 h 20 b>\nf>\n\n<f 181 -\n   pic 31 state 12 wait 3\n   <bp x 29.30119872526209 y 28.79651920190857 bp>\n   <w kind 1 x 43.77779948258218 y 39.055331510048525 weaponact 21 w>\n   <i kind 4 x 20 y 16 w 42 h 26 dvx 2 fall 70 vrest 20 bdefend 10 injury 30 i>\n   <i kind 4 x 40 y 35 w 27 h 29 dvx 2 fall 70 vrest 20 bdefend 10 injury 30 i>\n   <b kind 0 x 27 y 25 w 24 h 23 b>\nf>\n\n<f 182 -\n   pic 32 state 12 wait 3\n   <bp x 29.625771905318558 y 31.904352557110816 bp>\n   <w kind 1 x 51.19999790204919 y 41.1208037036435 weaponact 23 w>\n   <i kind 4 x 18 y 23 w 46 h 26 dvx 2 fall 70 vrest 20 bdefend 10 injury 30 i>\n   <b kind 0 x 32 y 27 w 20 h 18 b>\nf>\n\n<f 183 -\n   pic 33 state 12 wait 3\n   <w kind 1 x 45 y 42 weaponact 33 cover 1 w>\n   <i kind 4 x 37 y 23 w 33 h 27 dvx 2 fall 70 vrest 20 bdefend 10 injury 30 i>\n   <i kind 4 x 15 y 43 w 38 h 21 dvx 2 fall 70 vrest 20 bdefend 10 injury 30 i>\n   <b kind 0 x 27 y 35 w 27 h 21 b>\nf>\n\n<f 184 -\n   pic 34 state 12 wait 3 centery 77\n   <bp x 29.353407673173237 y 64.34448184526693 bp>\n   <w kind 1 x 50.71790734309482 y 79.66647331391574 weaponact 32 w>\nf>\n\n<f 185 -\n   pic 35 state 12 wait 3\n   <bp x 30.190230589916823 y 50.830624988374424 bp>\n   <w kind 1 x 42.150696657273585 y 74.69644233620875 weaponact 31 w>\nf>\n\n<f 186 -\n   pic 40 state 12 wait 3\n   <bp x 44.3164372178733 y 27.33384943352798 bp>\n   <w kind 1 x 38.345639099432866 y 53.21421790570382 weaponact 34 w>\n   <i kind 4 x 27 y 17 w 36 h 50 dvx 2 fall 70 vrest 20 bdefend 10 injury 30 i>\n   <b kind 0 x 36 y 29 w 25 h 23 b>\nf>\n\n<f 187 -\n   pic 41 state 12 wait 3\n   <bp x 51.38853076650684 y 42.65335136303321 bp>\n   <w kind 1 x 32.76090299281674 y 51.4072386275756 weaponact 20 w>\n   <i kind 4 x 38 y 11 w 26 h 46 dvx 2 fall 70 vrest 20 bdefend 10 injury 30 i>\n   <i kind 4 x 31 y 48 w 21 h 29 dvx 2 fall 70 vrest 20 bdefend 10 injury 30 i>\n   <b kind 0 x 33 y 32 w 24 h 26 b>\nf>\n\n<f 188 -\n   pic 42 state 12 wait 3\n   <bp x 56.74213190441054 y 51.00492542155155 bp>\n   <w kind 1 x 50.35173633117958 y 62.1625229218968 weaponact 22 w>\n   <i kind 4 x 19 y 34 w 58 h 23 dvx 2 fall 70 vrest 20 bdefend 10 injury 30 i>\n   <b kind 0 x 35 y 36 w 24 h 21 b>\nf>\n\n<f 189 -\n   pic 43 state 12 wait 3\n   <bp x 56.2976874599661 y 66.5604809771071 bp>\n   <w kind 1 x 50.35173633117958 y 73.27363403300791 weaponact 25 w>\n   <i kind 4 x 29 y 32 w 26 h 28 dvx 2 fall 70 vrest 20 bdefend 10 injury 30 i>\n   <i kind 4 x 42 y 50 w 31 h 28 dvx 2 fall 70 vrest 20 bdefend 10 injury 30 i>\n   <b kind 0 x 35 y 44 w 23 h 21 b>\nf>\n\n<f 190 -\n   pic 44 state 12 wait 3 centery 80\n   <bp x 57.4138808745262 y 81.81636069893024 bp>\n   <w kind 1 x 46.43042360707956 y 81.3016868465666 weaponact 24 w>\nf>\n\n<f 191 -\n   pic 45 state 12 wait 3\n   <bp x 56.74213190441054 y 57.67159208821822 bp>\n   <w kind 1 x 50.35173633117958 y 68.82918958856347 weaponact 25 w>\nf>\n\n<f 200 ice\n   pic 8 state 15 wait 2 next 201\n   <bp x 43.912716762528504 y 42.60857231578623 bp>\n   <w kind 1 x 29.40247817772082 y 57.20555950244316 weaponact 22 w>\n   <b kind 0 x 15 y 14 w 55 h 68 b>\nf>\n\n<f 201 -\n   pic 9 state 13 wait 90 next 202\n   <bp x 38.53029898360305 y 45.75368914524945 bp>\n   <w kind 1 x 34.10681134060306 y 65.13296217204937 weaponact 21 w>\n   <i kind 14 x 13 y 11 w 67 h 73 vrest 1 i>\n   <b kind 0 x 13 y 11 w 67 h 73 b>\nf>\n\n<f 202 -\n   pic 8 state 15 wait 1 next 182 dvx -4 dvy -3\n   <bp x 43.912716762528504 y 42.60857231578623 bp>\n   <w kind 1 x 29.40247817772082 y 57.20555950244316 weaponact 22 w>\n   <b kind 0 x 13 y 11 w 67 h 73 b>\nf>\n\n<f 203 fire\n   pic 108 state 18 wait 1 next 204\n   <w kind 1 x 44.30747217968979 y 50.468665539726494 weaponact 21 w>\n   <i kind 0 x 27 y 40 w 26 h 19 dvx -6 dvy -6 fall 70 vrest 10 bdefend 16 injury 30 effect 20 i>\n   <b kind 0 x 27 y 40 w 26 h 19 b>\nf>\n\n<f 204 -\n   pic 109 state 18 wait 1 next 203\n   <w kind 1 x 44.30747217968979 y 50.468665539726494 weaponact 21 w>\n   <i kind 0 x 27 y 40 w 26 h 19 dvx -6 dvy -6 fall 70 vrest 10 bdefend 16 injury 30 effect 20 i>\n   <b kind 0 x 27 y 40 w 26 h 19 b>\nf>\n\n<f 205 -\n   pic 110 state 18 wait 1 next 206\n   <w kind 1 x 46.541246537522575 y 49.398651965595555 weaponact 35 w>\n   <i kind 0 x 27 y 40 w 26 h 19 dvx -6 dvy -6 fall 70 vrest 10 bdefend 16 injury 30 effect 20 i>\n   <b kind 0 x 27 y 40 w 26 h 19 b>\nf>\n\n<f 206 -\n   pic 111 state 18 wait 1 next 205\n   <w kind 1 x 46.541246537522575 y 49.398651965595555 weaponact 35 w>\n   <i kind 0 x 27 y 40 w 26 h 19 dvx -6 dvy -6 fall 70 vrest 10 bdefend 16 injury 30 effect 20 i>\n   <b kind 0 x 27 y 40 w 26 h 19 b>\nf>\n\n<f 207 tired\n   pic 69 state 15 wait 2\n   <w kind 1 x 47 y 69 weaponact 22 w>\n   <b kind 0 x 49 y 33 w 22 h 37 b>\n   <b kind 0 x 33 y 52 w 28 h 35 b>\nf>\n\n<f 210 jump\n   pic 60 state 4 wait 1 next 211 centerx 47\n   <bp x 49.1008823727453 y 52.25512380471005 bp>\n   <w kind 1 x 53 y 72 weaponact 32 cover 1 w>\n   <b kind 0 x 27 y 33 w 36 h 52 b>\nf>\n\n<f 211 -\n   pic 61 state 4 wait 1 next 212 centerx 49\n   sound mp3/017\n   <bp x 51.1008823727453 y 52.92179047137672 bp>\n   <w kind 1 x 55 y 74 weaponact 32 cover 1 w>\n   <b kind 0 x 32 y 33 w 34 h 52 b>\nf>\n\n<f 212 -\n   pic 62 state 4 wait 1\n   <bp x 49.57555555555556 y 33.24 bp>\n   <w kind 1 x 53 y 45 weaponact 30 cover 1 w>\n   <b kind 0 x 33 y 8 w 23 h 65 b>\n   <b kind 0 x 23 y 34 w 48 h 17 b>\nf>\n\n<f 213 dash\n   pic 63 state 5 wait 8 next 216\n   <bp x 61.57204587947352 y 38.80926056988844 bp>\n   <w kind 1 x 54 y 49 weaponact 31 cover 1 w>\n   <b kind 0 x 48 y 10 w 23 h 33 b>\n   <b kind 0 x 33 y 34 w 21 h 33 b>\n   <b kind 0 x 23 y 53 w 27 h 21 b>\nf>\n\n<f 214 -\n   pic 64 state 5 wait 8 next 217\n   <bp x 39.54862866753014 y 34.01258503705709 bp>\n   <w kind 1 x 46 y 40 weaponact 31 cover 1 w>\n   <b kind 0 x 25 y 10 w 27 h 38 b>\n   <b kind 0 x 21 y 42 w 36 h 22 b>\nf>\n\n<f 215 crouch\n   pic 60 state 15 wait 2 next 999 centerx 47\n   sound mp3/012\n   <bp x 49.1008823727453 y 52.25512380471005 bp>\n   <w kind 1 x 54 y 76 weaponact 32 cover 1 w>\n   <b kind 0 x 30 y 33 w 36 h 51 b>\nf>\n\n<f 216 dash\n   pic 112 state 5 wait 2\n   <bp x 61.75827728849966 y 39.41043804145079 bp>\n   <w kind 1 x 50 y 45 weaponact 31 cover 1 w>\n   <b kind 0 x 40 y 13 w 27 h 27 b>\n   <b kind 0 x 21 y 35 w 39 h 37 b>\nf>\n\n<f 217 -\n   pic 113 state 5 wait 2\n   <bp x 39.693455486987766 y 33.848078337386184 bp>\n   <w kind 1 x 41 y 40 weaponact 31 cover 1 w>\n   <b kind 0 x 23 y 18 w 29 h 51 b>\nf>\n\n<f 218 stop_running\n   pic 114 state 15 wait 5 next 999 dvx 1\n   sound mp3/009\n   <bp x 50.09258202227103 y 39.345983759643644 bp>\n   <w kind 1 x 49 y 57 weaponact 31 cover 1 w>\n   <b kind 0 x 22 y 30 w 30 h 55 b>\n   <b kind 0 x 50 y 52 w 16 h 32 b>\nf>\n\n<f 219 crouch2\n   pic 60 state 15 wait 2 next 999 centerx 45\n   sound mp3/012\n   <bp x 49.1008823727453 y 52.25512380471005 bp>\n   <w kind 1 x 55 y 78 weaponact 32 cover 1 w>\n   <b kind 0 x 31 y 35 w 33 h 49 b>\nf>\n\n<f 220 injured\n   pic 120 state 11 wait 2 next 221 centerx 52\n   <bp x 58.560752861996406 y 43.66327764426981 bp>\n   <w kind 1 x 52 y 53 weaponact 31 cover 1 w>\n   <b kind 0 x 30 y 22 w 29 h 61 b>\nf>\n\n<f 221 -\n   pic 121 state 11 wait 3 next 999 centerx 47\n   <bp x 50.58681032340757 y 49.29981210644321 bp>\n   <w kind 1 x 53 y 54 weaponact 31 cover 1 w>\n   <b kind 0 x 37 y 21 w 27 h 63 b>\n   <b kind 0 x 27 y 42 w 26 h 42 b>\nf>\n\n<f 222 -\n   pic 123 state 11 wait 2 next 223\n   <bp x 27.19838402341337 y 37.41742966619866 bp>\n   <w kind 1 x 46 y 54 weaponact 31 cover 1 w>\n   <b kind 0 x 16 y 29 w 39 h 31 b>\n   <b kind 0 x 30 y 58 w 40 h 27 b>\nf>\n\n<f 223 -\n   pic 124 state 11 wait 3 next 999\n   <bp x 33.92189058362268 y 39.402748070058934 bp>\n   <w kind 1 x 47 y 53 weaponact 31 cover 1 w>\n   <b kind 0 x 17 y 28 w 40 h 37 b>\n   <b kind 0 x 32 y 61 w 36 h 24 b>\nf>\n\n<f 224 -\n   pic 130 state 11 wait 2 next 225 centerx 46\n   <bp x 41.8985460310879 y 32.59923670441245 bp>\n   <w kind 1 x 52 y 45 weaponact 30 cover 1 w>\n   <b kind 0 x 30 y 23 w 31 h 61 b>\nf>\n\n<f 225 -\n   pic 131 state 11 wait 3 next 999 centerx 49\n   <bp x 45.721522797847854 y 34.49926072579309 bp>\n   <w kind 1 x 55 y 48 weaponact 30 cover 1 w>\n   <b kind 0 x 29 y 23 w 35 h 63 b>\nf>\n\n<f 226 -\n   pic 120 state 16 wait 6 next 227 centerx 48\n   <bp x 58.560752861996406 y 43.66327764426981 bp>\n   <w kind 1 x 52 y 51 weaponact 31 cover 1 w>\n   <i kind 6 x 11 y 17 w 85 h 68 vrest 1 i>\n   <b kind 0 x 32 y 27 w 42 h 58 b>\nf>\n\n<f 227 -\n   pic 122 state 16 wait 6 next 228 centerx 41\n   <bp x 49.291429639060475 y 48.34931721551483 bp>\n   <w kind 1 x 54 y 52 weaponact 31 cover 1 w>\n   <i kind 6 x 11 y 17 w 85 h 68 vrest 1 i>\n   <b kind 0 x 33 y 29 w 39 h 57 b>\nf>\n\n<f 228 -\n   pic 121 state 16 wait 6 next 229 centerx 42\n   <bp x 50.58681032340757 y 49.29981210644321 bp>\n   <w kind 1 x 53 y 52 weaponact 31 cover 1 w>\n   <i kind 6 x 11 y 17 w 85 h 68 vrest 1 i>\n   <b kind 0 x 33 y 28 w 37 h 58 b>\nf>\n\n<f 229 -\n   pic 122 state 16 wait 6 next 999 centerx 42\n   <bp x 49.291429639060475 y 48.34931721551483 bp>\n   <w kind 1 x 54 y 51 weaponact 31 cover 1 w>\n   <i kind 6 x 11 y 17 w 85 h 68 vrest 1 i>\n   <b kind 0 x 34 y 31 w 37 h 53 b>\nf>\n\n<f 230 lying\n   pic 34 state 14 wait 30 next 219 centery 77\n   <bp x 29.353407673173237 y 64.34448184526693 bp>\n   <w kind 1 x 51.71790734309482 y 79.66647331391574 weaponact 32 w>\nf>\n\n<f 231 -\n   pic 44 state 14 wait 30 next 219 centery 80\n   <bp x 57.4138808745262 y 81.81636069893024 bp>\n   <w kind 1 x 48.43042360707956 y 81.3016868465666 weaponact 24 w>\nf>\n\n<f 232 throw_lying_man\n   pic 27 state 9 wait 3 next 233\n   <bp x 44.53670834964537 y 38.96496959566491 bp>\n   <c kind 1 x 33 y 14 vaction 135 dircontrol 1 c>\n   <w kind 1 x 47 y 53 weaponact 31 cover 1 w>\n   <b kind 0 x 23 y 20 w 36 h 65 b>\nf>\n\n<f 233 -\n   pic 28 state 9 wait 1 next 234 centerx 40\n   sound mp3/007\n   <c kind 1 x 77 y 58 vaction 181 throwvx 13 throwvy -7 throwvz 3 throwinjury 30 c>\n   <w kind 1 x 51 y 57 weaponact 32 cover 1 w>\n   <b kind 0 x 15 y 33 w 61 h 28 b>\n   <b kind 0 x 24 y 61 w 30 h 24 b>\nf>\n\n<f 234 -\n   pic 28 state 9 wait 4 next 999 centerx 40\n   <w kind 1 x 51 y 57 weaponact 32 cover 1 w>\n   <b kind 0 x 18 y 35 w 57 h 28 b>\n   <b kind 0 x 24 y 61 w 30 h 24 b>\nf>\n\n<f 235 transform\n   pic 90 state 9 wait 3 next 236 mp 150\n   sound mp3/063\n   <bp x 53.5874919036096 y 40.172935507380345 bp>\n   <c kind 1 x 66 y 44 vaction 130 hurtable 1 c>\n   <w kind 1 x 52 y 54 weaponact 31 cover 1 w>\n   <b kind 0 x 24 y 20 w 28 h 65 b>\nf>\n\n<f 236 -\n   pic 91 state 9 wait 3 next 237\n   <bp x 53.5874919036096 y 40.172935507380345 bp>\n   <c kind 1 x 66 y 44 vaction 130 hurtable 1 c>\n   <w kind 1 x 52 y 54 weaponact 31 cover 1 w>\n   <b kind 0 x 24 y 20 w 28 h 65 b>\nf>\n\n<f 237 -\n   pic 92 state 9 wait 3 next 238\n   <bp x 53.5874919036096 y 40.172935507380345 bp>\n   <c kind 1 x 66 y 44 vaction 130 hurtable 1 c>\n   <w kind 1 x 52 y 54 weaponact 31 cover 1 w>\n   <b kind 0 x 24 y 20 w 28 h 65 b>\nf>\n\n<f 238 -\n   pic 93 state 9 wait 3 next 239\n   sound mp3/061\n   <o kind 1 x 46 y 75 action 70 oid 204 o>\n   <bp x 53.5874919036096 y 40.172935507380345 bp>\n   <c kind 1 x 66 y 44 vaction 130 hurtable 1 c>\n   <w kind 1 x 52 y 54 weaponact 31 cover 1 w>\n   <b kind 0 x 24 y 20 w 28 h 65 b>\nf>\n\n<f 239 -\n   pic 93 state 9 wait 1 next 240\n   <bp x 53.5874919036096 y 40.172935507380345 bp>\n   <c kind 1 x 77 y 85 vaction 181 throwvx 8 throwvy -3 throwinjury -1 c>\n   <w kind 1 x 52 y 54 weaponact 31 cover 1 w>\n   <b kind 0 x 24 y 20 w 28 h 65 b>\nf>\n\n<f 240 -\n   pic 93 state 9 wait 1 next 999\n   <bp x 53.5874919036096 y 40.172935507380345 bp>\n   <w kind 1 x 52 y 54 weaponact 31 cover 1 w>\n   <b kind 0 x 24 y 20 w 28 h 65 b>\nf>\n\n<f 245 transform_b\n   pic 100 state 9 wait 1 next 246 centerx 46\n   <bp x 48.464444444444446 y 38.35111111111111 bp>\n   <w kind 1 x 51 y 54 weaponact 30 cover 1 w>\n   <b kind 0 x 26 y 23 w 43 h 62 b>\nf>\n\n<f 246 -\n   pic 101 state 9 wait 1 next 247 centerx 46\n   sound mp3/063\n   <o kind 1 x 46 y 75 action 70 oid 204 o>\n   <bp x 48.464444444444446 y 38.35111111111111 bp>\n   <w kind 1 x 51 y 54 weaponact 30 cover 1 w>\n   <b kind 0 x 26 y 23 w 43 h 62 b>\nf>\n\n<f 247 -\n   pic 102 state 9 wait 1 next 248 centerx 46\n   sound mp3/061\n   <bp x 48.464444444444446 y 38.35111111111111 bp>\n   <w kind 1 x 51 y 54 weaponact 30 cover 1 w>\n   <b kind 0 x 26 y 23 w 43 h 62 b>\nf>\n\n<f 248 -\n   pic 103 state 9 wait 2 next 999 centerx 46\n   <bp x 48.464444444444446 y 38.35111111111111 bp>\n   <w kind 1 x 51 y 54 weaponact 30 cover 1 w>\n   <b kind 0 x 26 y 23 w 43 h 62 b>\nf>\n\n<f 250 disappear\n   pic 85 state 15 wait 3 next 251 centerx 46 mp 350\n   <bp x 48.26 y 38.19777777777778 bp>\n   <w kind 1 x 51 y 54 weaponact 30 cover 1 w>\n   <b kind 0 x 26 y 23 w 43 h 62 b>\nf>\n\n<f 251 -\n   pic 84 state 15 wait 2 next 252 centerx 46\n   <bp x 48.26 y 38.19777777777778 bp>\n   <w kind 1 x 51 y 54 weaponact 30 cover 1 w>\n   <b kind 0 x 26 y 23 w 43 h 62 b>\nf>\n\n<f 252 -\n   pic 85 state 15 wait 2 next 253 centerx 46\n   <bp x 48.26 y 38.19777777777778 bp>\n   <w kind 1 x 51 y 54 weaponact 30 cover 1 w>\n   <b kind 0 x 26 y 23 w 43 h 62 b>\nf>\n\n<f 253 -\n   pic 84 state 15 wait 1 next 254 centerx 46\n   <bp x 48.26 y 38.19777777777778 bp>\n   <w kind 1 x 51 y 54 weaponact 30 cover 1 w>\n   <b kind 0 x 26 y 23 w 43 h 62 b>\nf>\n\n<f 254 -\n   pic 85 state 15 wait 1 next 255 centerx 46\n   <bp x 48.26 y 38.19777777777778 bp>\n   <w kind 1 x 51 y 54 weaponact 30 cover 1 w>\n   <b kind 0 x 26 y 23 w 43 h 62 b>\nf>\n\n<f 255 -\n   pic 84 state 15 wait 1 next 256 centerx 46\n   sound mp3/061\n   <bp x 48.26 y 38.19777777777778 bp>\n   <w kind 1 x 51 y 54 weaponact 30 cover 1 w>\n   <b kind 0 x 26 y 23 w 43 h 62 b>\nf>\n\n<f 256 -\n   pic 85 state 15 wait 1 next 257 centerx 46\n   <o kind 1 x 46 y 75 action 60 oid 204 o>\n   <bp x 48.26 y 38.19777777777778 bp>\n   <w kind 1 x 51 y 54 weaponact 30 cover 1 w>\n   <b kind 0 x 26 y 23 w 43 h 62 b>\nf>\n\n<f 257 -\n   pic 84 state 15 wait 1 next 1280 centerx 46\n   <bp x 48.26 y 38.19777777777778 bp>\n   <w kind 1 x 51 y 54 weaponact 30 cover 1 w>\n   <b kind 0 x 26 y 23 w 43 h 62 b>\nf>\n\n<f 260 +man\n   pic 85 state 15 wait 3 next 261 centerx 46 mp 350\n   <bp x 48.26 y 38.19777777777778 bp>\n   <w kind 1 x 51 y 54 weaponact 30 cover 1 w>\n   <b kind 0 x 26 y 23 w 43 h 62 b>\nf>\n\n<f 261 -\n   pic 84 state 15 wait 2 next 262 centerx 46\n   sound mp3/062\n   <bp x 48.26 y 38.19777777777778 bp>\n   <w kind 1 x 51 y 54 weaponact 30 cover 1 w>\n   <b kind 0 x 26 y 23 w 43 h 62 b>\nf>\n\n<f 262 -\n   pic 85 state 15 wait 2 next 263 centerx 46\n   <bp x 48.26 y 38.19777777777778 bp>\n   <w kind 1 x 51 y 54 weaponact 30 cover 1 w>\n   <b kind 0 x 26 y 23 w 43 h 62 b>\nf>\n\n<f 263 -\n   pic 84 state 15 wait 1 next 264 centerx 46\n   <bp x 48.26 y 38.19777777777778 bp>\n   <w kind 1 x 51 y 54 weaponact 30 cover 1 w>\n   <b kind 0 x 26 y 23 w 43 h 62 b>\nf>\n\n<f 264 -\n   pic 78 state 15 wait 1 next 265 centerx 46\n   <bp x 48.26 y 38.19777777777778 bp>\n   <w kind 1 x 51 y 54 weaponact 30 cover 1 w>\n   <b kind 0 x 26 y 23 w 43 h 62 b>\nf>\n\n<f 265 -\n   pic 79 state 15 wait 1 next 266 centerx 46\n   <bp x 48.26 y 38.19777777777778 bp>\n   <w kind 1 x 51 y 54 weaponact 30 cover 1 w>\n   <b kind 0 x 26 y 23 w 43 h 62 b>\nf>\n\n<f 266 -\n   pic 88 state 15 wait 1 next 267 centerx 46\n   <bp x 48.26 y 38.19777777777778 bp>\n   <w kind 1 x 51 y 54 weaponact 30 cover 1 w>\n   <b kind 0 x 26 y 23 w 43 h 62 b>\nf>\n\n<f 267 -\n   pic 86 state 15 wait 2 next 268 centerx 46\n   <bp x 48.26 y 38.19777777777778 bp>\n   <w kind 1 x 51 y 54 weaponact 30 cover 1 w>\n   <b kind 0 x 26 y 23 w 43 h 62 b>\nf>\n\n<f 268 -\n   pic 89 state 15 wait 1 next 269 centerx 46\n   <bp x 48.26 y 38.19777777777778 bp>\n   <w kind 1 x 51 y 54 weaponact 30 cover 1 w>\n   <b kind 0 x 26 y 23 w 43 h 62 b>\nf>\n\n<f 269 -\n   pic 87 state 15 wait 1 next 270 centerx 46\n   <bp x 48.26 y 38.19777777777778 bp>\n   <w kind 1 x 51 y 54 weaponact 30 cover 1 w>\n   <b kind 0 x 26 y 23 w 43 h 62 b>\nf>\n\n<f 270 -\n   pic 88 state 15 wait 1 next 271 centerx 46\n   <bp x 48.26 y 38.19777777777778 bp>\n   <w kind 1 x 51 y 54 weaponact 30 cover 1 w>\n   <b kind 0 x 26 y 23 w 43 h 62 b>\nf>\n\n<f 271 -\n   pic 79 state 15 wait 1 next 999 centerx 46\n   <o kind 1 x 45 y 84 oid 5 facing 20 o>\n   <bp x 48.26 y 38.19777777777778 bp>\n   <w kind 1 x 51 y 54 weaponact 30 cover 1 w>\n   <b kind 0 x 26 y 23 w 43 h 62 b>\nf>\n\n<f 273 jump_sword\n   pic 22 state 3 wait 1 next 274 centerx 36 centery 83\n   <bp x 65.5137545143159 y 55.18645971015323 bp>\n   <w kind 1 x 51 y 65 weaponact 32 cover 1 w>\n   <b kind 0 x 20 y 35 w 52 h 46 b>\nf>\n\n<f 274 -\n   pic 150 state 3 wait 1 next 275 dvx 13 dvy -7 centerx 45 centery 63\n   sound mp3/017\n   <bp x 68.51961050577849 y 33.940539940502646 bp>\n   <w kind 1 x 51 y 41 weaponact 32 cover 1 w>\n   <b kind 0 x 28 y 11 w 44 h 57 b>\nf>\n\n<f 275 -\n   pic 150 state 3 wait 2 next 276 centerx 45 centery 60\n   <bp x 68.51961050577849 y 33.940539940502646 bp>\n   <w kind 1 x 51 y 41 weaponact 32 cover 1 w>\n   <b kind 0 x 28 y 10 w 43 h 56 b>\nf>\n\n<f 276 -\n   pic 151 state 3 wait 1 next 277 centerx 27 centery 61\n   sound mp3/028\n   <bp x 48.92861304550895 y 33.98644597490677 bp>\n   <w kind 1 x 36 y 41 weaponact 32 cover 1 w>\n   <i kind 0 x 44 y 23 w 55 h 44 dvx 2 fall 60 vrest 15 bdefend 16 injury 35 effect 1 i>\n   <b kind 0 x 9 y 7 w 61 h 56 b>\nf>\n\n<f 277 -\n   pic 152 state 3 wait 1 next 278 centerx 28 centery 61\n   <bp x 52.35505325533708 y 35.16997260413854 bp>\n   <w kind 1 x 42 y 45 weaponact 32 cover 1 w>\n   <i kind 0 x 38 y 5 w 49 h 38 dvx 2 fall 60 vrest 15 bdefend 16 injury 35 effect 1 i>\n   <b kind 0 x 10 y 12 w 56 h 53 b>\nf>\n\n<f 278 -\n   pic 153 state 3 wait 1 next 279 centerx 53 centery 61\n   <bp x 77.13283103311485 y 36.28108371524965 bp>\n   <w kind 1 x 65 y 46 weaponact 32 cover 1 w>\n   <i kind 0 x 22 y 9 w 54 h 24 dvx 2 fall 60 vrest 15 bdefend 16 injury 35 effect 1 i>\n   <b kind 0 x 34 y 11 w 51 h 56 b>\nf>\n\n<f 279 -\n   pic 154 state 3 wait 1 next 280 centerx 49 centery 58\n   <bp x 73.13283103311485 y 34.16997260413854 bp>\n   <w kind 1 x 60 y 45 weaponact 32 cover 1 w>\n   <b kind 0 x 31 y 9 w 50 h 59 b>\nf>\n\n<f 280 -\n   pic 155 state 3 wait 1 next 281 centerx 38 centery 56\n   <bp x 62.13283103311487 y 34.61441704858299 bp>\n   <w kind 1 x 49 y 42 weaponact 32 cover 1 w>\n   <b kind 0 x 21 y 12 w 47 h 56 b>\nf>\n\n<f 281 -\n   pic 150 state 3 wait 7 next 999 centerx 46 centery 58\n   sound mp3/027\n   <bp x 68.51961050577849 y 33.940539940502646 bp>\n   <w kind 1 x 55 y 45 weaponact 32 cover 1 w>\n   <b kind 0 x 25 y 10 w 49 h 57 b>\nf>\n\n<f 285 punch\n   pic 10 state 3 wait 3 next 286 centerx 45 mp 100\n   <bp x 48.75061461791846 y 38.42940829813039 bp>\n   <w kind 1 x 51 y 56 weaponact 31 cover 1 w>\n   <b kind 0 x 28 y 20 w 31 h 63 b>\nf>\n\n<f 286 -\n   pic 11 state 3 wait 1 next 287 centerx 47\n   sound mp3/007\n   <bp x 51.18 y 38.59111111111111 bp>\n   <w kind 1 x 51 y 56 weaponact 31 cover 1 w>\n   <b kind 0 x 33 y 19 w 29 h 63 b>\nf>\n\n<f 287 -\n   pic 12 state 3 wait 1 next 288 centerx 45\n   <bp x 49.825838059315736 y 38.98216753134385 bp>\n   <w kind 1 x 51 y 56 weaponact 31 cover 1 w>\n   <b kind 0 x 31 y 21 w 30 h 64 b>\nf>\n\n<f 288 -\n   pic 13 state 3 wait 1 next 289 centerx 46\n   <o kind 1 x 80 y 62 action 40 dvx 17 dvy -3 oid 202 facing 50 o>\n   <bp x 51.45702584630638 y 39.20820242827308 bp>\n   <w kind 1 x 51 y 56 weaponact 31 cover 1 w>\n   <b kind 0 x 28 y 17 w 32 h 69 b>\nf>\n\n<f 289 -\n   pic 13 state 3 wait 3 next 999 centerx 46 hit_a 285\n   <bp x 51.45702584630638 y 39.20820242827308 bp>\n   <w kind 1 x 51 y 56 weaponact 31 cover 1 w>\n   <b kind 0 x 28 y 17 w 32 h 69 b>\nf>\n\n<f 295 transform\n   pic 103 state 500 wait 3 next 296 centerx 46\n   <bp x 48.464444444444446 y 38.35111111111111 bp>\n   <w kind 1 x 51 y 54 weaponact 30 cover 1 w>\n   <b kind 0 x 26 y 23 w 43 h 62 b>\nf>\n\n<f 296 -\n   pic 102 state 9 wait 2 next 297 centerx 46\n   sound mp3/063\n   <bp x 48.464444444444446 y 38.35111111111111 bp>\n   <w kind 1 x 51 y 54 weaponact 30 cover 1 w>\n   <b kind 0 x 26 y 23 w 43 h 62 b>\nf>\n\n<f 297 -\n   pic 101 state 9 wait 1 next 298 centerx 46\n   sound mp3/061\n   <o kind 1 x 46 y 75 action 70 oid 204 o>\n   <bp x 48.464444444444446 y 38.35111111111111 bp>\n   <w kind 1 x 51 y 54 weaponact 30 cover 1 w>\n   <b kind 0 x 26 y 23 w 43 h 62 b>\nf>\n\n<f 298 -\n   pic 100 state 501 wait 1 next 999 centerx 46\n   <bp x 48.464444444444446 y 38.35111111111111 bp>\n   <w kind 1 x 51 y 54 weaponact 30 cover 1 w>\n   <b kind 0 x 26 y 23 w 43 h 62 b>\nf>\n\n<f 399 dummy\n   pic 0 centerx 46\n   <bp x 48.464444444444446 y 38.35111111111111 bp>\n   <b kind 0 x 26 y 23 w 43 h 62 b>\nf>\n\n"
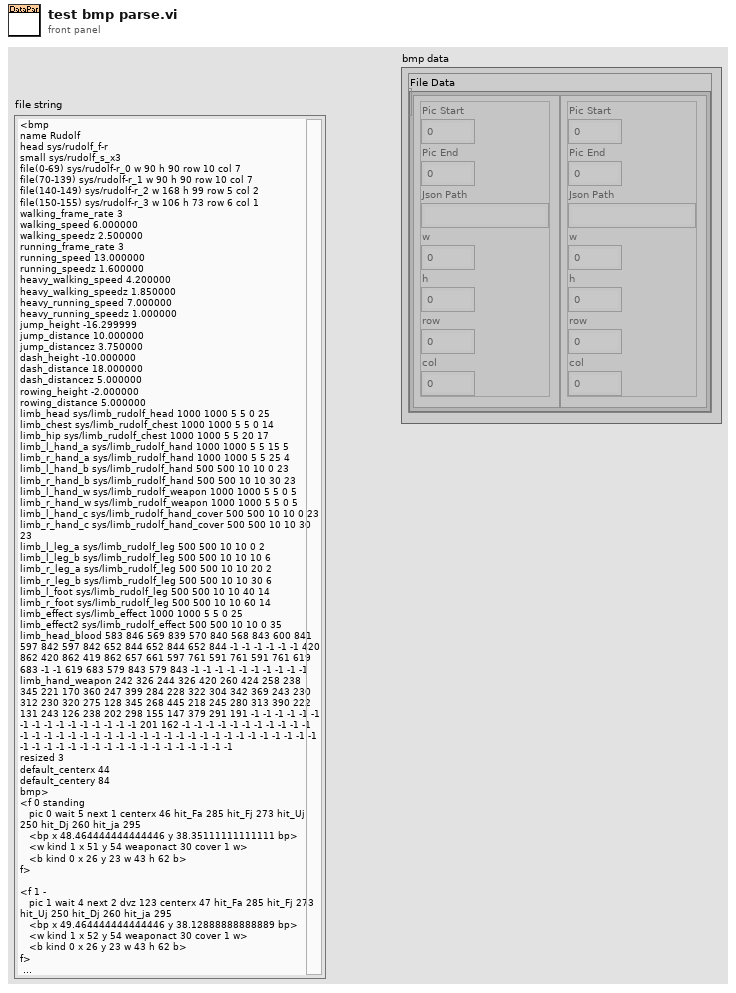
[diagram p1: front panel]
types:
  T1 = typedef "Data Parser.lvclass/Bmp data.ctl" = cluster{"File Data":cluster{"Pic Start":i32, "Pic End":i32, "Json Path":string, "w":i32, "h":i32, "row":i32, "col":i32}[]}
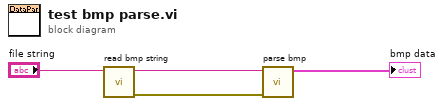
[diagram p0: block diagram]
diagram:
  n1 = call "read bmp string.vi"("file string"="file string") -> ("error out"=w2:errorcluster, "<bmp> string"=w3:string)  [unwired: 8 in, 1 out]
  n2 = call "parse bmp.vi"("error in (no error)"=w2, "<bmp> string"=w3) -> ("bmp data"=→"bmp data":T1)  [unwired: 8 in, 1 out]
